vi "Implement IIR Cascade Filter for N Specs and N Chan (CDB).vi"(7 "reset filter states":bool[](array[boolean]), 8 "error in (no error)":errorcluster, 10 "arrIIRFIlterCluster":T1(array[cluster]) {"Forward Coefficients" format="%0.4f"; "Reverse Coefficients" format="%0.4f"}, 11 "arrWaveforms":waveform(cdb)[](array[waveform])) -> (0 "error out":errorcluster, 3 "arrFilteredWaveforms":waveform(cdb)[](array[waveform]))   [LabVIEW 2020, in "NI_MAPro.lvlib"]
uses:
  NI_MAPro.lvlib
  NI_MABase.lvlib
  NI_AALBase.lvlib
panel:
  in  "shift register type":cdb[](array[numeric]) format="%0.2f"
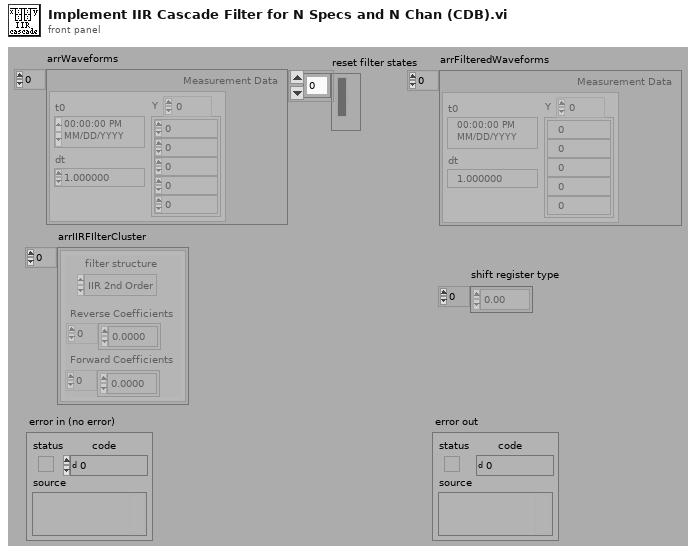
[diagram p1: front panel]
types:
  T1 = cluster{"filter structure":enum32{"IIR 2nd Order", "IIR 4th Order"}, "Reverse Coefficients":dbl[], "Forward Coefficients":dbl[]}[]
  T2 = cluster{"filter structure":enum32{"IIR 2nd Order", "IIR 4th Order"}, "Reverse Coefficients":dbl[], "Forward Coefficients":dbl[]}
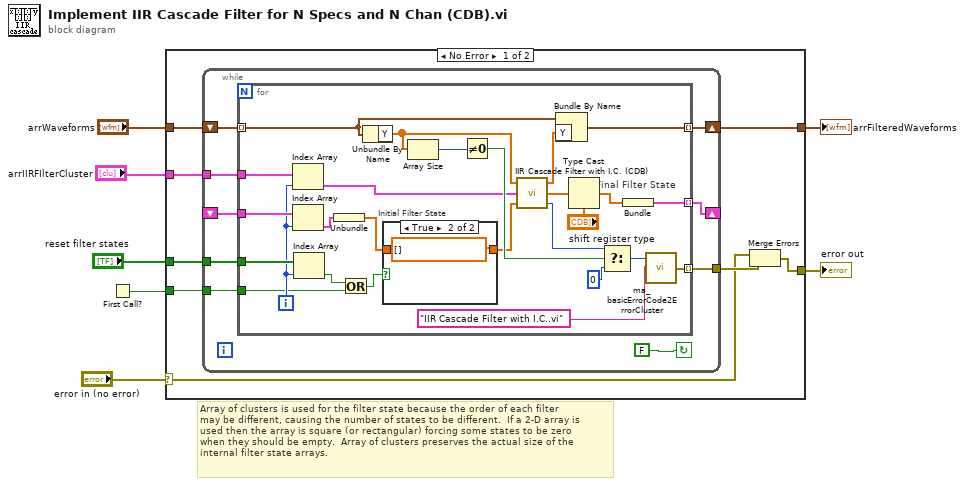
[diagram p0: block diagram]
diagram:
  # "Array of clusters is used for the filter state because the order of each filter \nmay be different, causing the number of states to be different.  If a 2-D array is \nused then the array is square (or rectangular) forcing some states to be zero\nwhen they should be empty.  Array of clusters preserves the actual size of the \ninternal filter state arrays."
  n1 = First Call?() -> (First Call?: T/F=w2:bool)
  n2 = case shown="No Error" "error in (no error)" {
    selector: "error in (no error)" -> [w10 w54]
    tunnel: [w12 w54] -> w6
    tunnel: "reset filter states" -> [w11 _]
    tunnel: "arrWaveforms" -> [w15 w53]
    tunnel: "arrIIRFIlterCluster" -> [w14 _]
    tunnel: [w9 w53] -> w3
    tunnel: w2 -> [w8 _]
    frame No Error {
      n3 = while {
        tunnel: w11 -> [w17]
        tunnel: [w18] -> w13
        tunnel: w14 -> [w20]
        shift-left: w15 -> [w22]
        shift-right: [w21] -> w9
        shift-left: _ -> [w24]
        shift-right: [w23] -> _
        tunnel: w8 -> [w16]
        stop <- FALSE continue-if-true
        n4 = for {
          tunnel: w24 -> [w45]
          tunnel: [w46] -> w23 mode=indexing
          tunnel: w22 -> [w38] mode=indexing
          tunnel: [w43] -> w21 mode=indexing
          tunnel: w20 -> [w48]
          tunnel: [w35] -> w18 mode=indexing
          tunnel: w17 -> [w37]
          tunnel: w16 -> [w25]
          i -> [w36]
          # "Final Filter State"
          # "Initial Filter State"
          n5 = Index Array(array=w48, index=w36) -> (element=w41:T2)
          n6 = Index Array(array=w45, index=w36) -> (element=w44:cluster{"shift register type":cdb[]})
          n7 = Index Array(array=w37, index=w36) -> (element=w27:bool)
          n8 = Unbundle(w44) -> ("shift register type"=w40:cdb[])
          n9 = Or(x=w27, y=w25) -> (x .or. y?=w26:bool)
          n10 = Unbundle By Name(w38) -> ("Y"=w28:cdb[])
          n11 = case shown="True" w26 {
            tunnel: w40 -> [w51 _]
            tunnel: [w51 cdb[] [] ("shift register type")] -> w39
            frame False {
            }
            frame True {
            }
          }
          n12 = Array Size(array=w28) -> (size(s)=w29:i32)
          n13 = Not Equal To 0?(x=w29) -> (x != 0?=w50:bool)
          n14 = call "IIR Cascade Filter with I.C. (CDB).vi"("Initial Filter State"=w39, "IIR Filter Cluster"=w41, "X"=w28) -> ("error"=w30:i32, "Final Filter State"=w42:cdb[], "Filtered X"=w34:cdb[])
          n15 = Bundle By Name(cluster=w38, "Y"=w34) -> (w43:waveform(cdb))
          n16 = Type Cast(type="shift register type", x=w42) -> (*(type *) &x=w47:cdb[])
          n17 = Select(t=w30, s=w50, f=0) -> (s? t:f=w31:i32)
          n18 = Bundle("shift register type"=w47) -> (w46:cluster{"shift register type":cdb[]})  [unwired: 1 in]
          n19 = call "ma_basicErrorCode2ErrorCluster.vi"("subVI name"="IIR Cascade Filter with I.C..vi", "Error Code"=w31) -> ("error out"=w35:errorcluster)  [unwired: 1 in]
        }
      }
      n20 = Merge Errors(w10, w13) -> (w12:errorcluster)
    }
    frame Error {
    }
  }
  "error out" <- w6
  "arrFilteredWaveforms" <- w3
